vi "To String.vi"(8 "error in (no error)":errorcluster, 11 "String Array in":refnum<class "String Array.lvclass">) -> (0 "error out":errorcluster, 2 "String":string)   [LabVIEW 2020, in "Data.lvlib" / "String Array.lvclass"]
doc: "Convert 'Generic Data in' to a string."
uses:
  String Array.lvclass
  String Array.lvclass/String Array.ctl
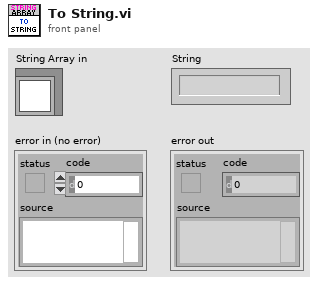
[diagram p1: front panel]
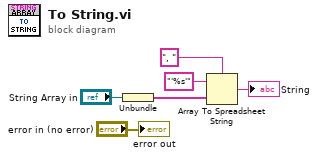
[diagram p0: block diagram]
diagram:
  n1 = Unbundle("String Array in") -> (w4:string[])
  n2 = Array To Spreadsheet String(delimiter (Tab)=", ", array=w4, 3:"'%s'" ("format string")) -> (spreadsheet string=→"String":string)
  "error out" <- "error in (no error)"
